vi "Create Function String (Frequency).vi"(8 "error in (no error)":errorcluster, 9 "Element/Wiring Unit (1: 1)":i32(ring)=1 items=["Null", "1", "2", "3", "4", "5", "6", "Sigma A", "Sigma B", "Sigma C"], 10 "Function (0: Frequency U)":i32(ring) items=["Frequency U", "Frequency I", "Frequency PLL1", "Frequency PLL2"], 11 "VISA resource name":refnum<visa-resource-name>) -> (0 "error out":errorcluster, 2 "Function String":string, 3 "VISA resource name out":refnum<visa-resource-name>)   [LabVIEW 2021, in "Yokogawa WT1800 Series.lvlib"]
doc: "Create a frequency function string.\n\n<b>Note:</b>\nOn models with the add-on frequency measurement (/FQ) option, \nall input elements can be measured simultaneously, so it is not \nnecessary to use this VI."
uses:
  <instrlib>/Yokogawa WT1800 Series/Yokogawa WT1800 Series.lvlib
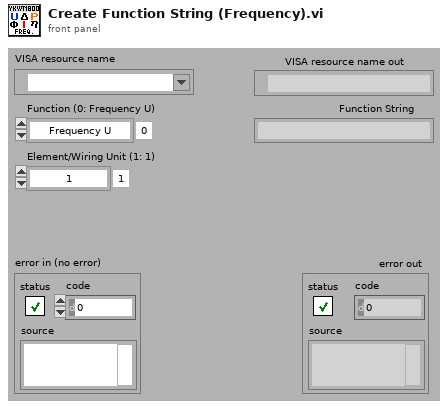
[diagram p1: front panel]
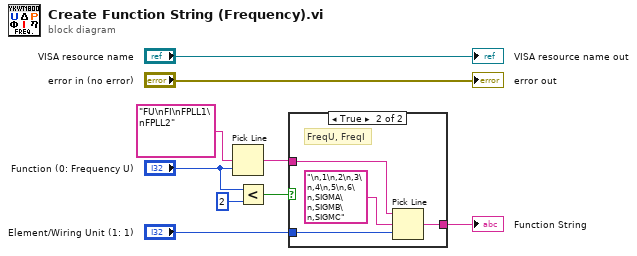
[diagram p0: block diagram]
diagram:
  n1 = Pick Line ("ライン選択")(multi-line string="FU\nFI\nFPLL1\nFPLL2" ("複数行文字列"), line index="Function (0: Frequency U)") -> (output string=w7:string)  [unwired: 1 in]
  n2 = Less?(x="Function (0: Frequency U)", y=2) -> (x < y?=w3:bool)
  n3 = case shown="True" w3 {
    tunnel: w7 -> [w10 w13]
    tunnel: "Element/Wiring Unit (1: 1)" -> [_ w12]
    tunnel: [w10 w11] -> w4
    frame False {
      # "Freq PLL1, Freq PLL2"
    }
    frame True {
      # "FreqU, FreqI"
      n4 = Pick Line ("ライン選択")(string ("")=w13, multi-line string="\n,1\n,2\n,3\n,4\n,5\n,6\n,SIGMA\n,SIGMB\n,SIGMC" ("複数行文字列"), line index=w12) -> (output string=w11:string)
    }
  }
  "Function String" <- w4
  "VISA resource name out" <- "VISA resource name"
  "error out" <- "error in (no error)"
